vi "get_control_in_Memory.vi"(2 "error in (no error)":errorcluster, 3 "Control Name":string, 5 "VI Name":string="Client with Signaling") -> (1 "error out 2":errorcluster, 4 "Value":variant)   [LabVIEW 2025]
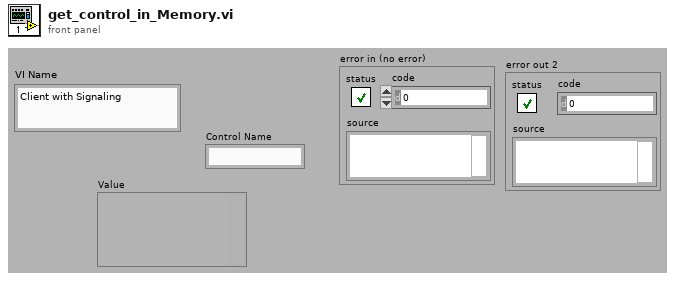
[diagram p1: front panel]
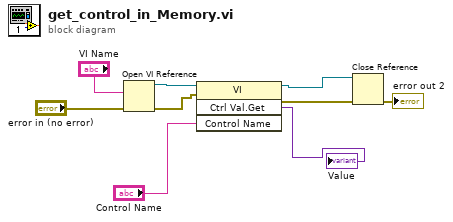
[diagram p0: block diagram]
diagram:
  n1 = Open VI Reference(vi path="VI Name", error in (no error)="error in (no error)") -> (vi reference=w9:refnum<vi>, error out=w3:errorcluster)  [unwired: 4 in]
  n2 = invoke class="VI" method="Ctrl Val.Get"(reference=w9, error in=w3, "Control Name"="Control Name") -> (reference out=w6:refnum<vi>, error out=w5:errorcluster, "Get Control Value Variant"=→"Value":variant)  [unwired: 1 in, 1 out]
  n3 = Close Reference(reference=w6, error in (no error)=w5) -> (error out=→"error out 2":errorcluster)
